vi "NGCode.vi"(8 "error in (no error)":errorcluster, 11 "Test Data":string[][](table)) -> (0 "error out":errorcluster, 3 "NG CODE OUT":string)   [LabVIEW 2018]
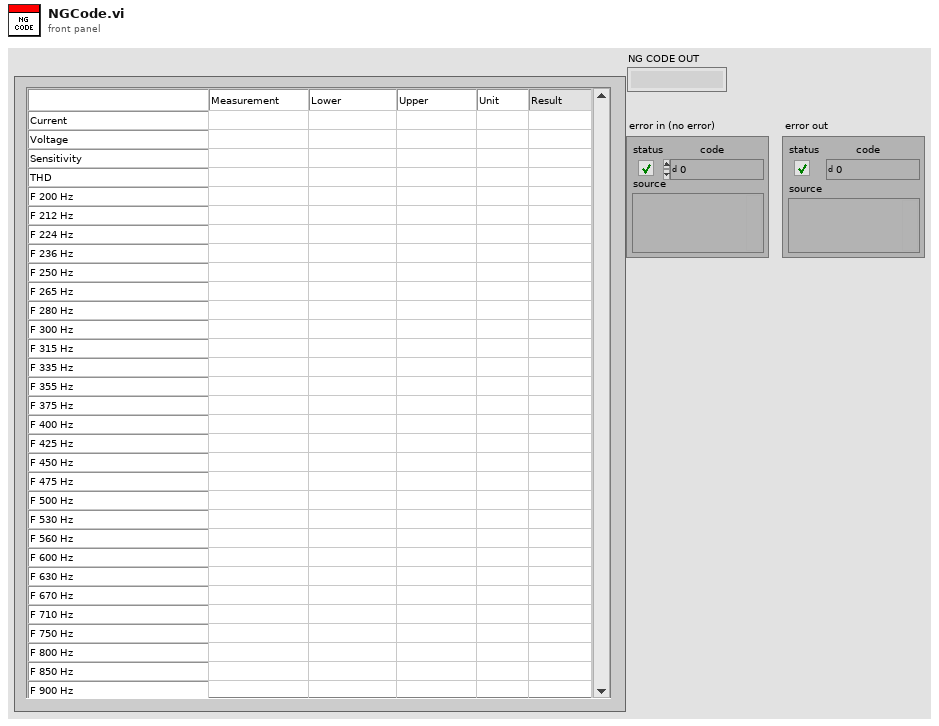
[diagram p1: front panel]
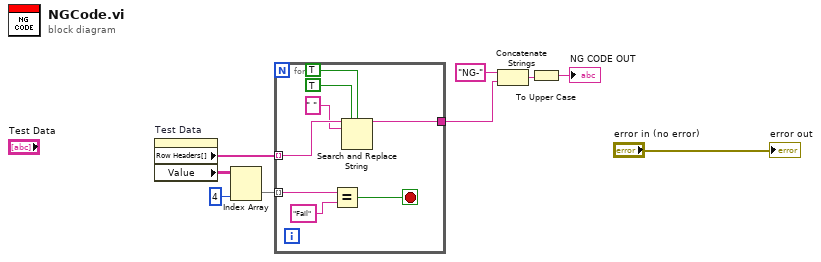
[diagram p0: block diagram]
diagram:
  n1 = property on="Test Data" class="Tbl (strict)"() -> ("Row Headers[]"=w9:string[], "Value"=w8:string[][])  [unwired: 2 in, 2 out]
  n2 = Index Array(array=w8, index (col)=4 ("disabled index (col)")) -> (element=w6:string[])  [unwired: 1 in]
  n3 = for {
    tunnel: w9 -> [w14] mode=indexing
    tunnel: w6 -> [w17] mode=indexing
    tunnel: [w10] -> w3
    stop <- w15 stop-if-true
    n4 = Equal?(x=w17, y="Fail") -> (x = y?=w15:bool)
    n5 = Search and Replace String(replace all?=TRUE ("replace all? (F)"), case sensitive?=TRUE ("ignore case? (F)"), input string=w14, search string=" ") -> (result string=w10:string)  [unwired: 4 in, 3 out]
  }
  n6 = Concatenate Strings("NG-", w3) -> (w2:string)
  n7 = To Upper Case(1:w2) -> (0:→"NG CODE OUT":string)
  "error out" <- "error in (no error)"
